vi "fp display engine.vi"(7 "channel data in":sgl[][][](array[numeric]), 10 "Image Refs In":T1[](array[typedef]), 11 "DisplayRefsIn(generic class)":refnum<vi>[](array[refnum])) -> ()   [LabVIEW 2012]
uses:
  <vilib>/vision/Image Controls.llb/IMAQ Image.ctl
  Custom Controls/MAIN Image panel tab Control type def.ctl
  Custom Controls/Ch selector.ctl
  GFG/GFGfpRefGet.vi
  GFG/GFGbooleanGet.vi
  <vilib>/vision/NI_Vision_Development_Module.lvlib
  GFG/GFG library.lvlib
panel:
  in  "ROI colors":u32[](array[colorbox])=[6618880, 16716362, 16860, 16776793, 16750848, 16448250, 16716530, 9567230, 16764108, 7340212, 32639, 0, 13816530, 8421376, 8421631, 7171459, 6618880, 16716362, 16860, 16776793, 16750848, 16448250, 16716530, 9567230, 16764108, 7340212, 32639, 0, 13816530, 8421376, 8421631, 7171459, 6618880, 16716362, 16860, 16776793, 16750848, 16448250, 16716530, 9567230, 16764108, 7340212, 32639, 0, 13816530, 8421376, 8421631, 7171459, 6618880, 16716362, 16860, 16776793, 16750848, 16448250, 16716530, 9567230, 16764108, 7340212, 32639, 0, 13816530, 8421376, 8421631, 7171459, 6618880, 16716362, 16860, 16776793, 16750848, 16448250, 16716530, 9567230, 16764108, 7340212, 32639, 0, 13816530, 8421376, 8421631, 7171459, 6618880, 16716362, 16860, 16776793, 16750848, 16448250, 16716530, 9567230, 16764108, 7340212, 32639, 0, 13816530, 8421376, 8421631, 7171459, 6618880, 16716362, 16860, 16776793, 16750848, 16448250, 16716530, 9567230, 16764108, 7340212, 32639, 0, 13816530, 8421376, 8421631, 7171459, 6618880, 16716362, 16860, 16776793, 16750848, 16448250, 16716530, 9567230, 16764108, 7340212, 32639, 0, 13816530, 8421376, 8421631, 7171459, 6618880, 16716362, 16860, 16776793, 16750848, 16448250, 16716530, 9567230, 16764108, 7340212, 32639, 0, 13816530, 8421376, 8421631, 7171459, 6618880, 16716362, 16860, 16776793, 16750848, 16448250, 16716530, 9567230, 16764108, 7340212, 32639, 0, 13816530, 8421376, 8421631, 7171459, 6618880, 16716362, 16860, 16776793, 16750848, 16448250, 16716530, 9567230, 16764108, 7340212, 32639, 0, 13816530, 8421376, 8421631, 7171459, 6618880, 16716362, 16860, 16776793, 16750848, 16448250, 16716530, 9567230, 16764108, 7340212, 32639, 0, 13816530, 8421376, 8421631, 7171459, 6618880, 16716362, 16860, 16776793, 16750848, 16448250, 16716530, 9567230, 16764108, 7340212, 32639, 0, 13816530, 8421376, 8421631, 7171459, 6618880, 16716362, 16860, 16776793, 16750848, 16448250, 16716530, 9567230, 16764108, 7340212, 32639, 0, 13816530, 8421376, 8421631, 7171459, 6618880, 16716362, 16860, 16776793, 16750848, 16448250, 16716530, 9567230, 16764108, 7340212, 32639, 0, 13816530, 8421376, 8421631, 7171459, 6618880, 16716362, 16860, 16776793, 16750848, 16448250, 16716530, 9567230, 16764108, 7340212, 32639, 0, 13816530, 8421376, 8421631, 7171459, 6618880, 16716362, 16860, 16776793, 16750848, 16448250, 16716530, 9567230, 16764108, 7340212, 32639, 0, 13816530, 8421376, 8421631, 7171459, 6618880, 16716362, 16860, 16776793, 16750848, 16448250, 16716530, 9567230, 16764108, 7340212, 32639, 0, 13816530, 8421376, 8421631, 7171459, 6618880, 16716362, 16860, 16776793, 16750848, 16448250, 16716530, 9567230, 16764108, 7340212, 32639, 0, 13816530, 8421376, 8421631, 7171459, 6618880, 16716362, 16860, 16776793, 16750848, 16448250, 16716530, 9567230, 16764108, 7340212, 32639, 0, 13816530, 8421376, 8421631, 7171459, 6618880, 16716362, 16860, 16776793, 16750848, 16448250, 16716530, 9567230, 16764108, 7340212, 32639, 0, 13816530, 8421376, 8421631, 7171459, 6618880, 16716362, 16860, 16776793, 16750848, 16448250, 16716530, 9567230, 16764108, 7340212, 32639, 0, 13816530, 8421376, 8421631, 7171459, 6618880, 16716362, 16860, 16776793, 16750848, 16448250, 16716530, 9567230, 16764108, 7340212, 32639, 0, 13816530, 8421376, 8421631, 7171459, 6618880, 16716362, 16860, 16776793, 16750848, 16448250, 16716530, 9567230, 16764108, 7340212, 32639, 0, 13816530, 8421376, 8421631, 7171459, 6618880, 16716362, 16860, 16776793, 16750848, 16448250, 16716530, 9567230, 16764108, 7340212, 32639, 0, 13816530, 8421376, 8421631, 7171459]
  out "error out":errorcluster
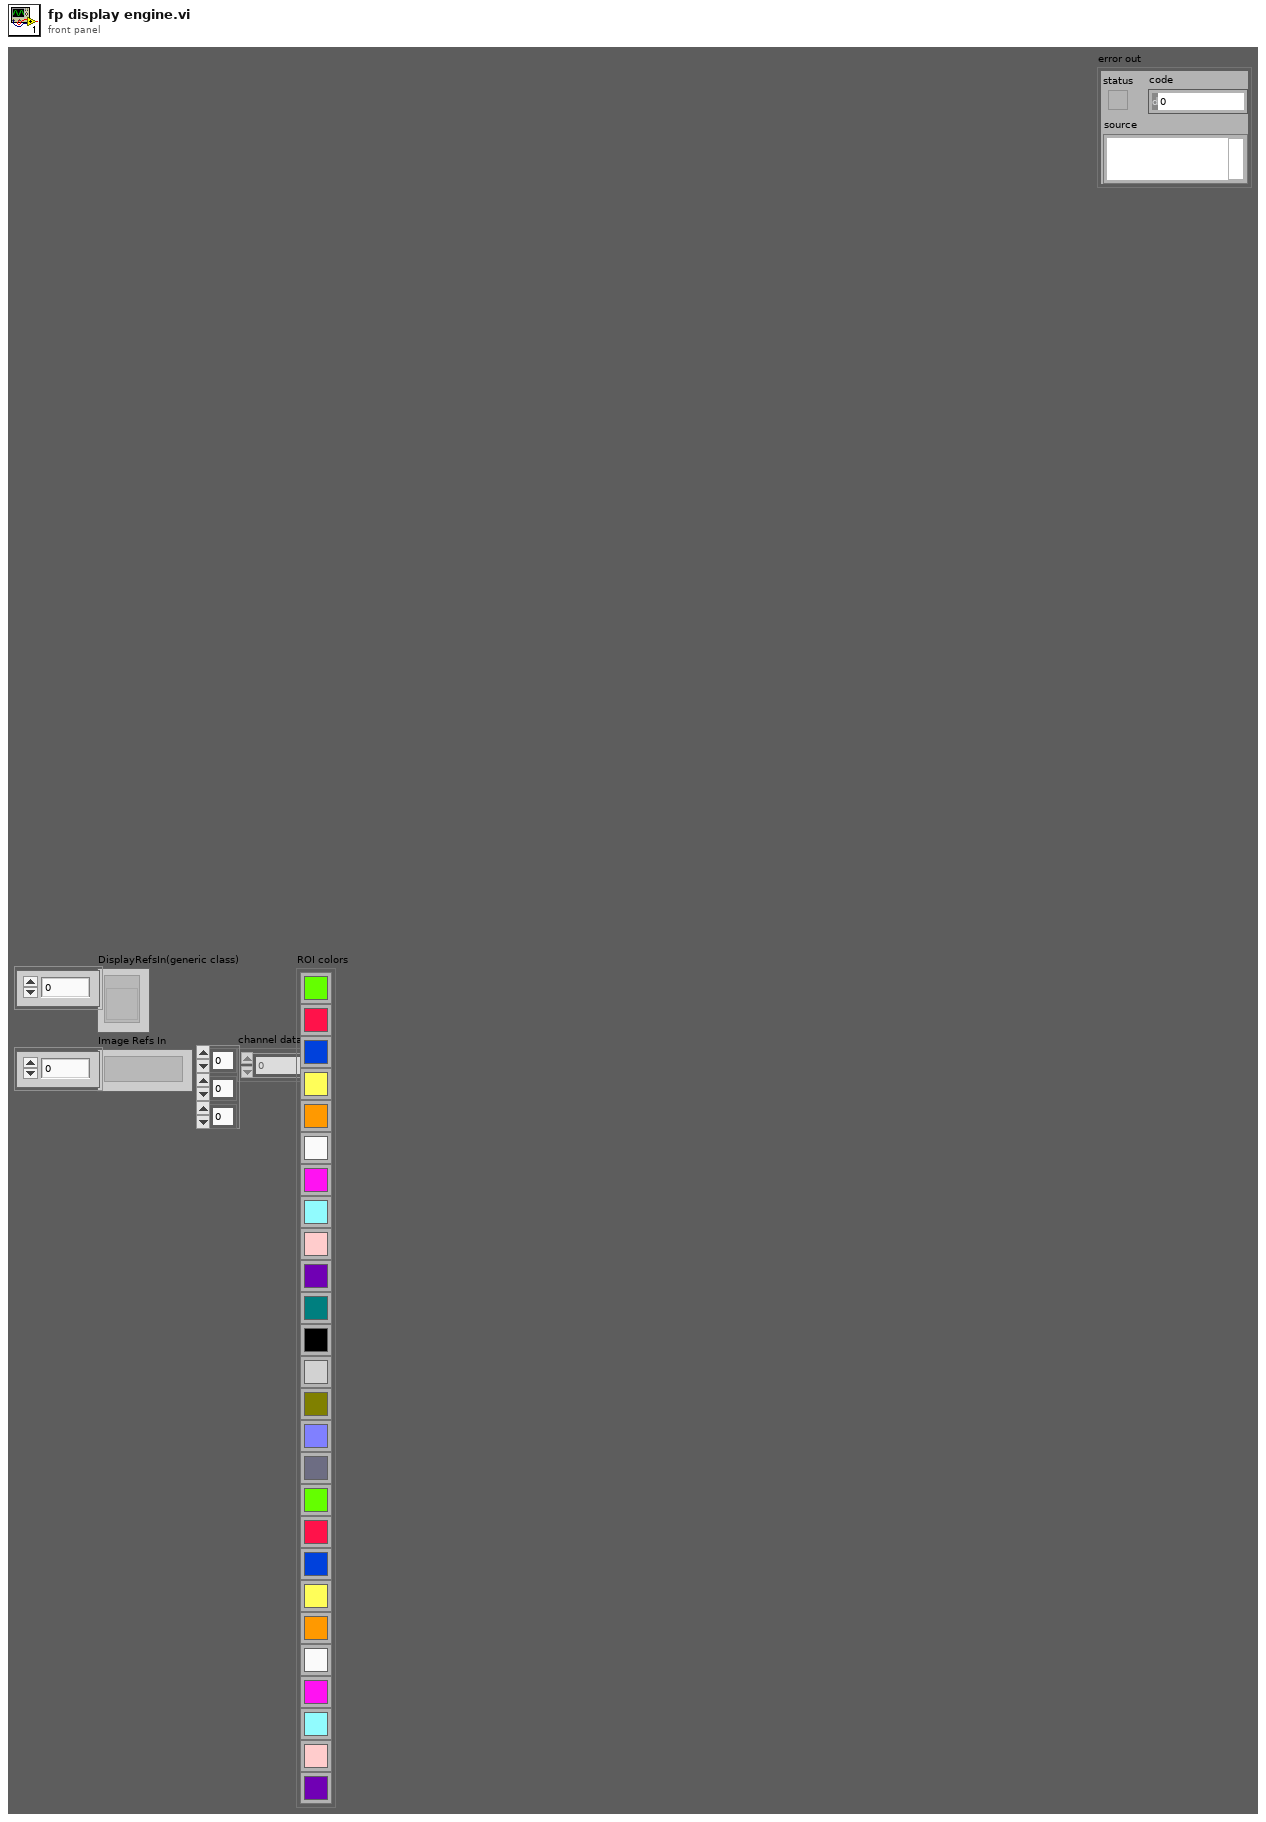
[diagram p1: front panel]
types:
  T1 = typedef "IMAQ Image.ctl" = refnum<image>
  T2 = typedef "MAIN Image panel tab Control type def.ctl" = enum32{"Channel 1", "Channel 2", "Channel 3", "Channel 4", "all channels", "RGB overlay", "ROI", "arbitrary line scan"}
  T3 = enum32{"Channel 1", "Channel 2", "Channel 3", "Channel 4", "Channel 5", "all channels", "RGB overlay", "ROI", "arbitrary line scan"}
  T4 = typedef "Ch selector.ctl" = enum16{"none", "Ch 1", "Ch 2", "Ch 3", "Ch 4", "Ch 5"}
  T5 = typedef "Image Type" = u32
  T6 = cluster{"Global Rectangle":i32[], "Contours":cluster{"Contour Type":u32, "ROI Type":u32, "Points":i32[]}[]}
  T7 = typedef "ROI Descriptor" = cluster{"Global Rectangle":i32[], "Contours":cluster{"ID":enum32{"External", "Internal"}, "Type":u32, "Coordinates":i32[]}[]}
  T8 = cluster{"WaveformChartRef":refnum<vi>, "DigitalRef":refnum<vi>, "ArrayRef":refnum<vi>, "TabControlRef":refnum<vi>, "EnumRef":refnum<vi>, "RingRef":refnum<vi>, "BooleanRef":refnum<vi>, "KnobRef":refnum<vi>, "SlideRef":refnum<vi>, "PathRef":refnum<vi>, "StringRef":refnum<vi>, "ComboBox":refnum<vi>, "WaveformGraphRef":refnum<vi>}
  T9 = cluster{"Mean Value":sgl, "Standard Variation":sgl, "Minimal Value":sgl, "Maximal Value":sgl, "Area (calibrated)":sgl, "Area (pixels)":i32, "%":sgl}[]
  T10 = cluster{"Mean Value":sgl, "Standard Variation":sgl, "Minimal Value":sgl, "Maximal Value":sgl, "Area (calibrated)":sgl, "Area (pixels)":i32, "%":sgl}
  T11 = cluster{"Contour Type":u32, "ROI Type":u32, "Points":i32[]}[]
  T12 = cluster{"Starting Value":sgl, "Incremental Value":sgl, "Histogram":u32[]}
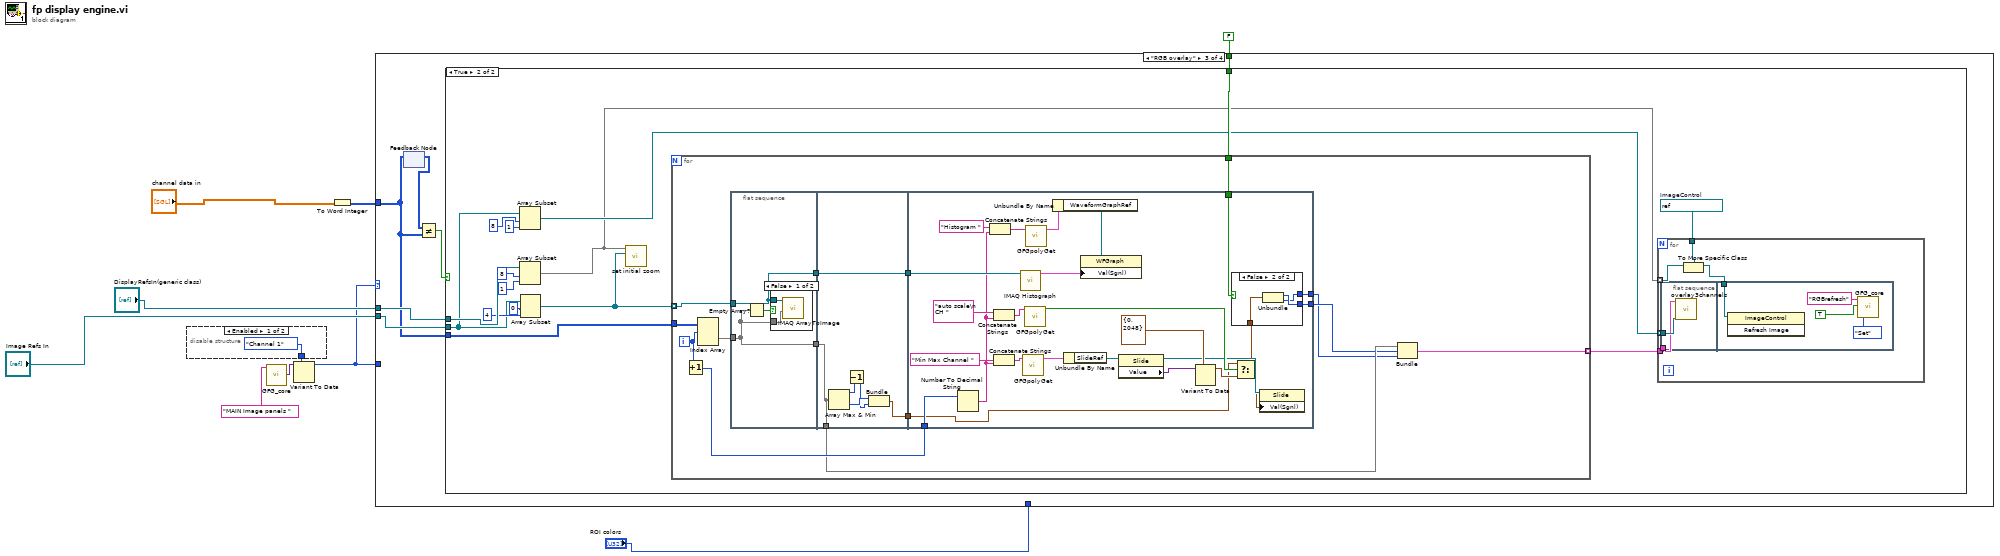
[diagram p0: block diagram]
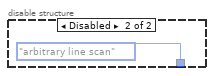
[diagram p2: hidden frame]
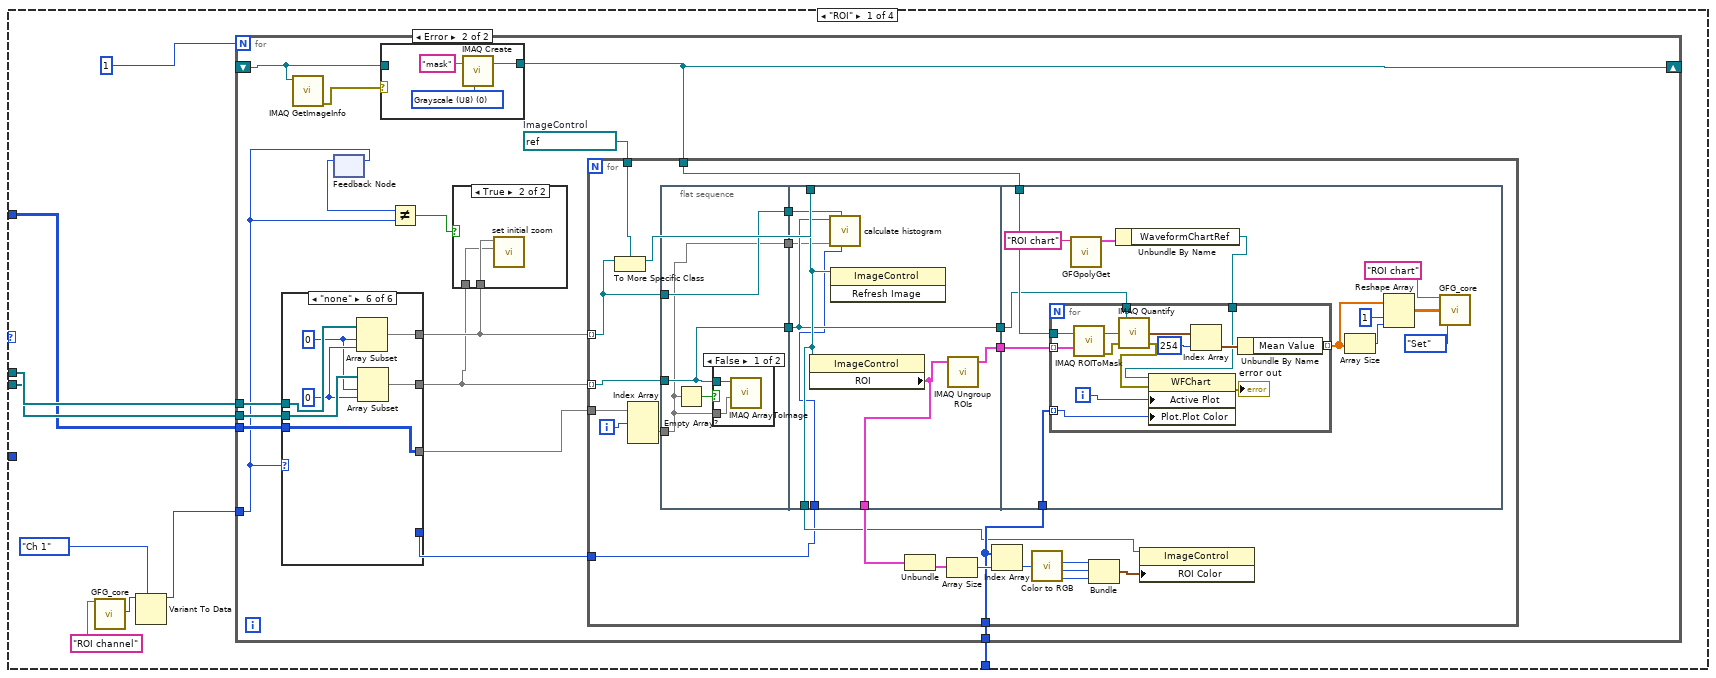
[diagram p3: hidden frame]
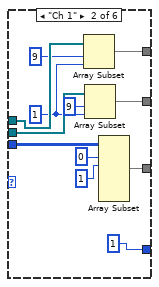
[diagram p7: hidden frame]
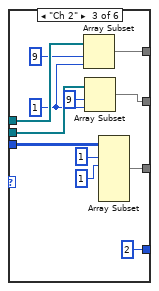
[diagram p8: hidden frame]
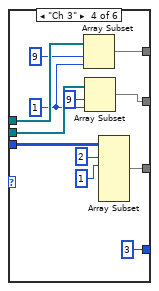
[diagram p9: hidden frame]
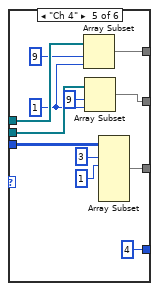
[diagram p10: hidden frame]
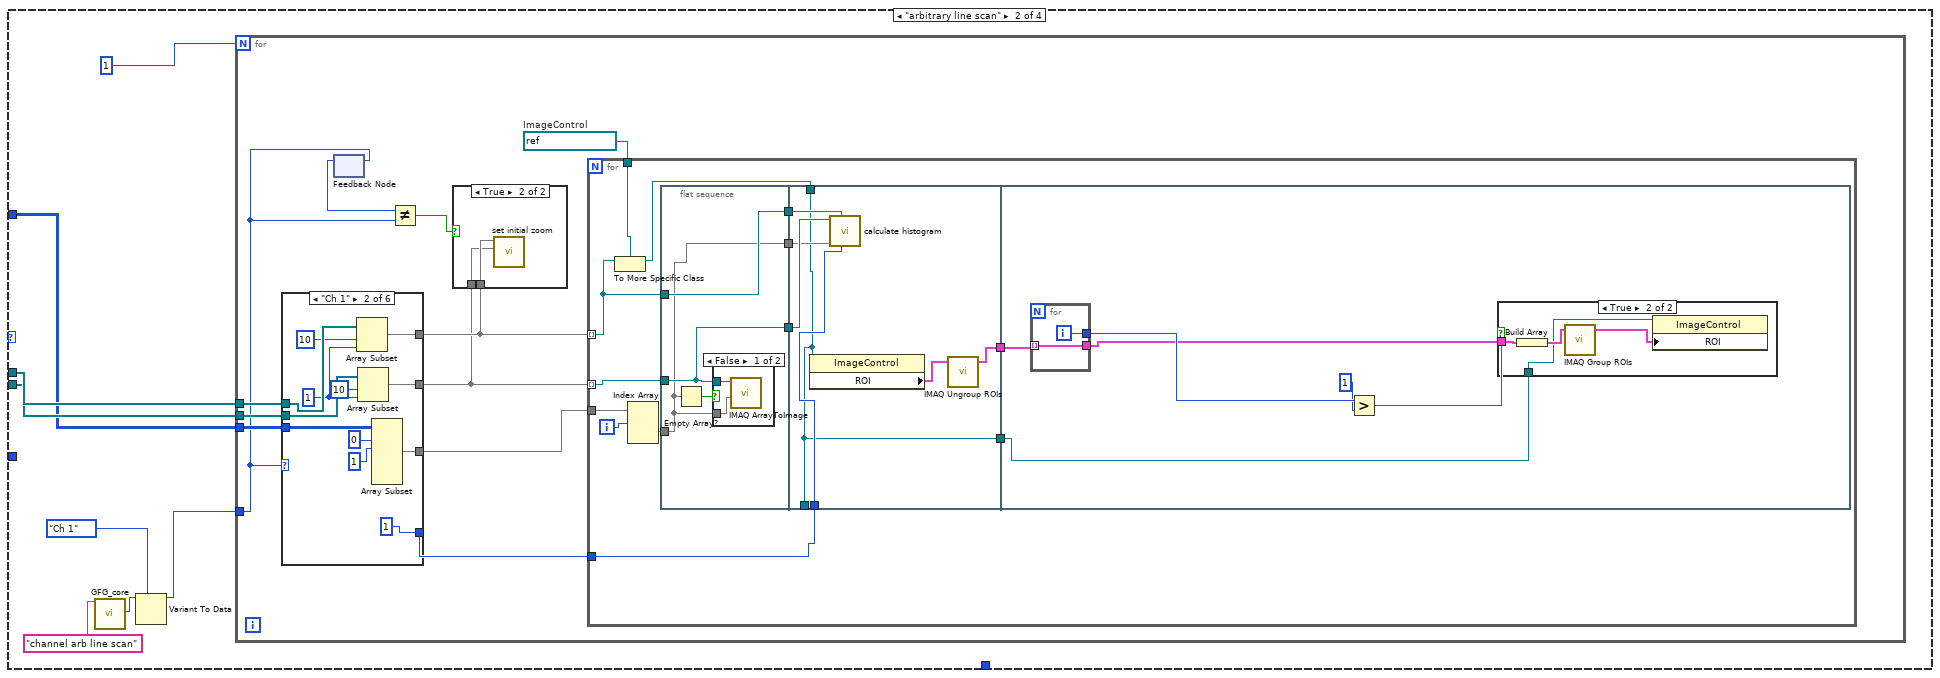
[diagram p12: hidden frame]
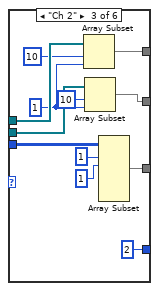
[diagram p15: hidden frame]
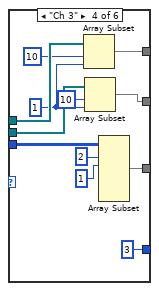
[diagram p16: hidden frame]
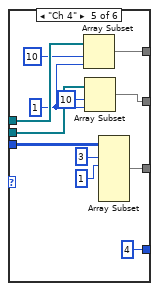
[diagram p17: hidden frame]
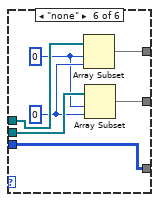
[diagram p18: hidden frame]
diagram:
  n1 = disable-structure shown="Enabled" {
    disable-tunnel: [MAIN_Image_panel_tab_Control_type_def."Channel 1" ("MAIN Image panels") T3."arbitrary line scan" ("MAIN Image panels")] -> w8
    frame Enabled {
    }
    frame Disabled {
    }
  }
  n2 = call "GFG_core.vi"("Variable Name in"="MAIN Image panels ") -> ("Variant Out"=w10:variant)  [unwired: 12 in, 6 out]
  n3 = Variant To Data(type=w8, Variant=w10) -> (data=w4:T2)  [unwired: 1 in, 1 out]
  n4 = To Word Integer(number="channel data in") -> (16bit integer=w3:i16[][][])
  n5 = case shown="\"RGB overlay\"" w4 {
    tunnel: w4 -> [_ _ _ w365]
    tunnel: "DisplayRefsIn(generic class)" -> [w20 w168 w281 w368]
    tunnel: "Image Refs In" -> [w19 w167 w279 w367]
    tunnel: w3 -> [w18 w166 w276 w366]
    tunnel: FALSE -> [_ _ w280 w363]
    tunnel: "ROI colors" -> [w14 _ _ _]
    frame "ROI" {
      n6 = call "GFG_core.vi"("Variable Name in"="ROI channel") -> ("Variant Out"=w16:variant)  [unwired: 12 in, 6 out]
      n7 = Variant To Data(type=Ch_selector."Ch 1" ("ROI channel"), Variant=w16) -> (data=w15:T4)  [unwired: 1 in, 1 out]
      n8 = for {
        N: 1 -> [_]
        tunnel: w20 -> [w35]
        tunnel: w19 -> [w34]
        tunnel: w18 -> [w33]
        tunnel: w15 -> [w30]
        shift-right: [w27] -> _
        shift-left: _ -> [w26]
        tunnel: w14 -> [w24]
        w32 = refnum<vi> refnum  # ImageControl
        n9 = case shown="\"none\"" w30 {
          tunnel: w35 -> [_ w53 w65 w77 w89 w96]
          tunnel: w34 -> [_ w54 w66 w78 w90 w97]
          tunnel: [_ w50 w62 w74 w86 w93] -> w22
          tunnel: [_ w49 w61 w73 w85 w92] -> w29
          tunnel: w33 -> [_ w48 w58 w70 w82 w91]
          tunnel: [_ w45 w57 w69 w81 w91] -> w36
          tunnel: [_ 1 ("length") 2 ("length") 3 ("length") 4 ("length") _] -> w23
          frame Default {
          }
          frame "Ch 1" {
            w52 = 1 ("length")
            n10 = Array Subset(array=w53, index=9, length=w52) -> (w49:refnum<vi>[])
            n11 = Array Subset(array=w54, index=9, length=w52) -> (w50:T1[])
            n12 = Array Subset(array=w48, index (dim 0)=0 ("index"), length (dim 0)=1 ("length")) -> (w45:i16[][][])  [unwired: 4 in]
          }
          frame "Ch 2" {
            w64 = 1 ("length")
            n13 = Array Subset(array=w65, index=9, length=w64) -> (w61:refnum<vi>[])
            n14 = Array Subset(array=w66, index=9, length=w64) -> (w62:T1[])
            n15 = Array Subset(array=w58, index (dim 0)=1 ("index"), length (dim 0)=1 ("length")) -> (w57:i16[][][])  [unwired: 4 in]
          }
          frame "Ch 3" {
            w75 = 1 ("index")
            n16 = Array Subset(array=w77, index=9, length=w75) -> (w73:refnum<vi>[])
            n17 = Array Subset(array=w78, index=9, length=w75) -> (w74:T1[])
            n18 = Array Subset(array=w70, index (dim 0)=2 ("index"), length (dim 0)=1 ("length")) -> (w69:i16[][][])  [unwired: 4 in]
          }
          frame "Ch 4" {
            w88 = 1 ("index")
            n19 = Array Subset(array=w89, index=9, length=w88) -> (w85:refnum<vi>[])
            n20 = Array Subset(array=w90, index=9, length=w88) -> (w86:T1[])
            n21 = Array Subset(array=w82, index (dim 0)=3 ("index"), length (dim 0)=1 ("length")) -> (w81:i16[][][])  [unwired: 4 in]
          }
          frame "none" {
            w94 = 0 ("index")
            w95 = 0 ("length")
            n22 = Array Subset(array=w96, index=w94, length=w95) -> (w92:refnum<vi>[])
            n23 = Array Subset(array=w97, index=w94, length=w95) -> (w93:T1[])
          }
        }
        n24 = call "IMAQ GetImageInfo"("Image"=w26) -> ("error out"=w25:errorcluster)  [unwired: 3 in, 7 out]
        n25 = feedback-in #1(w30) -> ()
        n26 = feedback #1() -> (w31:T4)  [unwired: 1 in]
        n27 = case shown="Error" w25 {
          tunnel: [w37 w38] -> w27
          tunnel: w26 -> [w37 _]
          frame No Error {
          }
          frame Error {
            w39 = T5 0 items=["Grayscale (U8)", "Grayscale (I16)", "Grayscale (SGL)", "Complex (CSG)", "RGB (U32)", "HSL (U32)", "RGB (U64)"] ("Image Type")
            n28 = call "IMAQ Create"("Image Name"="mask", "Image Type"=w39) -> ("New Image"=w38:T1)  [unwired: 3 in, 1 out]
          }
        }
        n29 = Not Equal?(x=w31, y=w30) -> (x != y?=w28:bool)
        n30 = case shown="True" w28 {
          tunnel: w29 -> [_ w42]
          tunnel: w22 -> [_ w41]
          frame False {
          }
          frame True {
            n31 = call "set initial zoom.vi"("Image Refs In"=w41, "DisplayRefsIn(generic class)"=w42) -> ()  [unwired: 10 in]
          }
        }
        n32 = for {
          tunnel: w29 -> [w100] mode=indexing
          tunnel: w22 -> [w119] mode=indexing
          tunnel: w36 -> [w121]
          tunnel: w32 -> [w118]
          tunnel: w27 -> [w103]
          tunnel: w24 -> [w106]
          tunnel: w23 -> [w98]
          i -> [w116]
          n33 = To More Specific Class(target class=w118, reference=w100) -> (specific class reference=w117:refnum<vi>)  [unwired: 1 in, 1 out]
          n34 = Index Array(array=w121, index (dim 0)=w116) -> (element=w120:i16[][])  [unwired: 2 in]
          n35 = flat-sequence {
            tunnel: w120 -> [w122]
            tunnel: w119 -> [w124]
            tunnel: [w124] -> w104
            tunnel: [w123] -> w101
            tunnel: w100 -> [w123]
            tunnel: [w122] -> w99
            tunnel: w117 -> [w132]
            tunnel: [w134] -> w109
            tunnel: [w133] -> w107
            tunnel: [w130] -> w105
            tunnel: w104 -> [w130]
            tunnel: [w132] -> w102
            tunnel: w101 -> [w131]
            tunnel: w99 -> [w129]
            tunnel: w98 -> [w128]
            tunnel: w107 -> [w144]
            tunnel: w106 -> [w143]
            tunnel: w105 -> [w135]
            tunnel: w103 -> [w136]
            frame #0 {
              n36 = Empty Array?(array=w122) -> (empty?=w125:bool)
              n37 = case shown="False" w125 {
                tunnel: w124 -> [w127 _]
                tunnel: w122 -> [w126 _]
                frame False {
                  n38 = call "IMAQ ArrayToImage"("Image Pixels (I16)"=w126, "Image"=w127) -> ()  [unwired: 8 in, 2 out]
                }
                frame True {
                }
              }
            }
            frame #1 {
              n39 = property class="ImageControl"(reference=w132) -> ("ROI"=w134:T6)  [unwired: 1 in, 2 out]
              n40 = call "calculate histogram.vi"("channel no."=w128, "Image Ctrl Ref (as generic class)"=w131, "Image Array"=w129, "Image"=w130) -> ()  [unwired: 8 in]
              n41 = invoke class="ImageControl" method="Refresh Image"(reference=w132) -> ()  [unwired: 2 in, 3 out]
              n42 = call "IMAQ Ungroup ROIs"("ROI Descriptor"=w134) -> ("ROI Descriptors out"=w133:T7[])  [unwired: 3 in, 1 out]
            }
            frame #2 {
              n43 = call-poly "GFGpolyGet.vi"("Variable Name in"="ROI chart") -> ("output cluster"=w138:T8)  [unwired: 9 in, 1 out]
              n44 = Unbundle By Name(w138) -> ("WaveformChartRef"=w137:refnum<vi>)
              n45 = for {
                tunnel: w135 -> [w161]
                tunnel: w144 -> [w155] mode=indexing
                tunnel: [w157] -> w147 mode=indexing
                tunnel: w136 -> [w154]
                tunnel: w143 -> [w151] mode=indexing
                tunnel: w137 -> [w150]
                i -> [w152]
                n46 = call "IMAQ ROIToMask"("ROI Descriptor"=w155, "Image"=w154) -> ("error out"=w149:errorcluster, "Image Out"=w156:T1)  [unwired: 4 in, 1 out]
                n47 = call "IMAQ Quantify"("error in (no error)"=w149, "Image Mask"=w156, "Image"=w161) -> ("error out"=w148:errorcluster, "Region Reports"=w160:T9)  [unwired: 1 out]
                n48 = property on="Property Node" class="WFChart"(reference=w150, error in=w148, "Active Plot"=w152, "Plot.Plot Color"=w151) -> (error out=→"error out":errorcluster)  [unwired: 1 out]
                n49 = Index Array(array=w160, index=254) -> (element=w158:T10)
                n50 = Unbundle By Name(w158) -> ("Mean Value"=w157:sgl)
              }
              n51 = Array Size(array=w147) -> (size(s)=w146:i32)
              n52 = Reshape Array(w147, 1 ("dimension size"), w146) -> (w141:sgl[][])
              n53 = call "GFG_core.vi"("Variable Name in"="ROI chart", "Variant in"=w141, "Action"=enum16{"Init", "Set", "Get"}."Set") -> ()  [unwired: 10 in, 7 out]
            }
          }
          n54 = Unbundle(w109) -> ("Contours"=w114:T11)  [unwired: 1 out]
          n55 = Array Size(array=w114) -> (size(s)=w115:i32)
          n56 = Index Array(array=w106, index=w115) -> (element=w110:u32)
          n57 = call <vilib>:"Color to RGB.vi"("Color"=w110) -> ("R"=w111:u8, "G"=w112:u8, "B"=w113:u8)  [unwired: 1 out]
          n58 = Bundle("R"=w111, "G"=w112, "B"=w113) -> (w108:cluster{"R":u8, "G":u8, "B":u8})  [unwired: 1 in]
          n59 = property class="ImageControl"(reference=w102, "ROI Color"=w108) -> ()  [unwired: 1 in, 2 out]
        }
      }
    }
    frame "arbitrary line scan" {
      n60 = call "GFG_core.vi"("Variable Name in"="channel arb line scan") -> ("Variant Out"=w164:variant)  [unwired: 12 in, 6 out]
      n61 = Variant To Data(type=Ch_selector."Ch 1" ("ROI channel"), Variant=w164) -> (data=w163:T4)  [unwired: 1 in, 1 out]
      n62 = for {
        N: 1 -> [_]
        tunnel: w168 -> [w179]
        tunnel: w167 -> [w178]
        tunnel: w166 -> [w177]
        tunnel: w163 -> [w174]
        w176 = refnum<vi> refnum  # ImageControl
        n63 = case shown="\"Ch 1\"" w174 {
          tunnel: w179 -> [_ w193 w205 w217 w229 w236]
          tunnel: w178 -> [_ w194 w206 w218 w230 w237]
          tunnel: [_ w190 w202 w214 w226 w233] -> w170
          tunnel: [_ w189 w201 w213 w225 w232] -> w173
          tunnel: w177 -> [_ w188 w198 w210 w222 w231]
          tunnel: [_ w185 w197 w209 w221 w231] -> w180
          tunnel: [_ 1 ("length") 2 ("length") 3 ("length") 4 ("length") _] -> w171
          frame Default {
          }
          frame "Ch 1" {
            w192 = 1 ("length")
            n64 = Array Subset(array=w193, index=10, length=w192) -> (w189:refnum<vi>[])
            n65 = Array Subset(array=w194, index=10, length=w192) -> (w190:T1[])
            n66 = Array Subset(array=w188, index (dim 0)=0 ("index"), length (dim 0)=1 ("length")) -> (w185:i16[][][])  [unwired: 4 in]
          }
          frame "Ch 2" {
            w204 = 1 ("length")
            n67 = Array Subset(array=w205, index=10, length=w204) -> (w201:refnum<vi>[])
            n68 = Array Subset(array=w206, index=10, length=w204) -> (w202:T1[])
            n69 = Array Subset(array=w198, index (dim 0)=1 ("index"), length (dim 0)=1 ("length")) -> (w197:i16[][][])  [unwired: 4 in]
          }
          frame "Ch 3" {
            w215 = 1 ("index")
            n70 = Array Subset(array=w217, index=10, length=w215) -> (w213:refnum<vi>[])
            n71 = Array Subset(array=w218, index=10, length=w215) -> (w214:T1[])
            n72 = Array Subset(array=w210, index (dim 0)=2 ("index"), length (dim 0)=1 ("length")) -> (w209:i16[][][])  [unwired: 4 in]
          }
          frame "Ch 4" {
            w228 = 1 ("index")
            n73 = Array Subset(array=w229, index=10, length=w228) -> (w225:refnum<vi>[])
            n74 = Array Subset(array=w230, index=10, length=w228) -> (w226:T1[])
            n75 = Array Subset(array=w222, index (dim 0)=3 ("index"), length (dim 0)=1 ("length")) -> (w221:i16[][][])  [unwired: 4 in]
          }
          frame "none" {
            w234 = 0 ("index")
            w235 = 0 ("length")
            n76 = Array Subset(array=w236, index=w234, length=w235) -> (w232:refnum<vi>[])
            n77 = Array Subset(array=w237, index=w234, length=w235) -> (w233:T1[])
          }
        }
        n78 = feedback-in #2(w174) -> ()
        n79 = feedback #2() -> (w175:T4)  [unwired: 1 in]
        n80 = Not Equal?(x=w175, y=w174) -> (x != y?=w172:bool)
        n81 = case shown="True" w172 {
          tunnel: w173 -> [_ w182]
          tunnel: w170 -> [_ w181]
          frame False {
          }
          frame True {
            n82 = call "set initial zoom.vi"("Image Refs In"=w181, "DisplayRefsIn(generic class)"=w182) -> ()  [unwired: 10 in]
          }
        }
        n83 = for {
          tunnel: w173 -> [w241] mode=indexing
          tunnel: w170 -> [w248] mode=indexing
          tunnel: w180 -> [w250]
          tunnel: w176 -> [w247]
          tunnel: w171 -> [w239]
          i -> [w245]
          n84 = To More Specific Class(target class=w247, reference=w241) -> (specific class reference=w246:refnum<vi>)  [unwired: 1 in, 1 out]
          n85 = Index Array(array=w250, index (dim 0)=w245) -> (element=w249:i16[][])  [unwired: 2 in]
          n86 = flat-sequence {
            tunnel: w249 -> [w251]
            tunnel: w248 -> [w253]
            tunnel: [w253] -> w243
            tunnel: [w252] -> w242
            tunnel: w241 -> [w252]
            tunnel: [w251] -> w240
            tunnel: w246 -> [w258]
            tunnel: [w263] -> w244
            tunnel: w243 -> [w261]
            tunnel: [w258] -> _
            tunnel: w242 -> [w262]
            tunnel: w240 -> [w260]
            tunnel: w239 -> [w259]
            tunnel: [w258] -> w238
            tunnel: w244 -> [w269]
            tunnel: w238 -> [w268]
            frame #0 {
              n87 = Empty Array?(array=w251) -> (empty?=w254:bool)
              n88 = case shown="False" w254 {
                tunnel: w253 -> [w256 _]
                tunnel: w251 -> [w255 _]
                frame False {
                  n89 = call "IMAQ ArrayToImage"("Image Pixels (I16)"=w255, "Image"=w256) -> ()  [unwired: 8 in, 2 out]
                }
                frame True {
                }
              }
            }
            frame #1 {
              n90 = property class="ImageControl"(reference=w258) -> ("ROI"=w257:T6)  [unwired: 1 in, 2 out]
              n91 = call "calculate histogram.vi"("channel no."=w259, "Image Ctrl Ref (as generic class)"=w262, "Image Array"=w260, "Image"=w261) -> ()  [unwired: 8 in]
              n92 = call "IMAQ Ungroup ROIs"("ROI Descriptor"=w257) -> ("ROI Descriptors out"=w263:T7[])  [unwired: 3 in, 1 out]
            }
            frame #2 {
              n93 = for {
                tunnel: w269 -> [w275] mode=indexing
                tunnel: [w275] -> w264
                tunnel: [w274] -> w267
                i -> [w274]
              }
              n94 = Greater?(x=w267, y=1) -> (0:w265:bool)
              n95 = case shown="True" w265 {
                tunnel: w264 -> [_ w273]
                tunnel: w268 -> [_ w270]
                frame False {
                }
                frame True {
                  n96 = Build Array(w273) -> (w272:T7[])
                  n97 = call "IMAQ Group ROIs"("ROI Descriptors"=w272) -> ("ROI Descriptor out"=w271:T7)  [unwired: 3 in, 1 out]
                  n98 = property class="ImageControl"(reference=w270, "ROI"=w271) -> ()  [unwired: 1 in, 2 out]
                }
              }
            }
          }
        }
      }
    }
    frame "RGB overlay" {
      n99 = feedback #3() -> (w278:i16[][][])  [unwired: 1 in]
      n100 = feedback-in #3(w276) -> ()
      n101 = Not Equal?(x=w278, y=w276) -> (x != y?=w277:bool)
      n102 = case shown="True" w277 {
        tunnel: w281 -> [_ w296]
        tunnel: w276 -> [_ w295]
        tunnel: w280 -> [_ w294]
        tunnel: w279 -> [_ w287]
        frame False {
        }
        frame True {
          w282 = refnum<vi> refnum  # ImageControl
          n103 = Array Subset(array=w287, index=8, length=1) -> (w286:T1[])
          n104 = Array Subset(array=w296, index=8, length=1) -> (w283:refnum<vi>[])
          n105 = Array Subset(array=w287, index=0, length=4) -> (w284:T1[])
          n106 = call "set initial zoom.vi"("Image Refs In"=w284, "DisplayRefsIn(generic class)"=w283) -> ()  [unwired: 10 in]
          n107 = for {
            tunnel: w284 -> [w319] mode=indexing
            tunnel: w295 -> [w321]
            tunnel: w294 -> [w312]
            tunnel: [w308] -> w285 mode=indexing
            i -> [w316]
            n108 = Increment(x=w316) -> (x+1=w314:i32)
            n109 = Index Array(array=w321, index (dim 0)=w316) -> (element=w320:i16[][])  [unwired: 2 in]
            n110 = flat-sequence {
              tunnel: w320 -> [w322]
              tunnel: w319 -> [w323]
              tunnel: [w323] -> w317
              tunnel: [w322] -> w315
              tunnel: [w332] -> w318
              tunnel: w317 -> [w332]
              tunnel: w315 -> [w327]
              tunnel: [w330] -> w313
              tunnel: [w327] -> w311
              tunnel: w318 -> [w351]
              tunnel: w314 -> [w350]
              tunnel: w313 -> [w338]
              tunnel: w312 -> [w333]
              tunnel: [w335] -> w309
              tunnel: [w334] -> w310
              frame #0 {
                n111 = Empty Array?(array=w322) -> (empty?=w324:bool)
                n112 = case shown="False" w324 {
                  tunnel: w323 -> [w326 _]
                  tunnel: w322 -> [w325 _]
                  frame False {
                    n113 = call "IMAQ ArrayToImage"("Image Pixels (I16)"=w325, "Image"=w326) -> ()  [unwired: 8 in, 2 out]
                  }
                  frame True {
                  }
                }
              }
              frame #1 {
                n114 = Array Max & Min(array=w327) -> (max value=w331:i16, min value=w329:i16)  [unwired: 2 out]
                n115 = Decrement(x=w331) -> (x-1=w328:i16)
                n116 = Bundle(w329, w328) -> (w330:cluster{i16, i16})  [unwired: 1 in]
              }
              frame #2 {
                n117 = Number To Decimal String(number=w350) -> (decimal integer string=w345:string)  [unwired: 1 in]
                n118 = Concatenate Strings("Histogram " ("string"), w345) -> (w353:string)
                n119 = Concatenate Strings("auto scale\n      CH " ("Variable Name in"), w345) -> (w348:string)
                n120 = Concatenate Strings("Min Max Channel " ("Variable Name in"), w345) -> (w336:string)
                n121 = call "IMAQ Histograph"("Image"=w351) -> ("Histogram Graph"=w356:T12)  [unwired: 7 in, 3 out]
                n122 = call-poly "GFGpolyGet.vi"("Variable Name in"=w336) -> ("output cluster"=w347:T8)  [unwired: 9 in, 1 out]
                n123 = call-poly "GFGpolyGet.vi"("Variable Name in"=w348) -> ("Boolean"=w341:bool)  [unwired: 10 in]
                n124 = call-poly "GFGpolyGet.vi"("Variable Name in"=w353) -> ("output cluster"=w354:T8)  [unwired: 9 in, 1 out]
                n125 = Unbundle By Name(w354) -> ("WaveformGraphRef"=w355:refnum<vi>)
                n126 = Unbundle By Name(w347) -> ("SlideRef"=w344:refnum<vi>)
                n127 = property class="WFGraph"(reference=w355, "Val(Sgnl)"=w356) -> ()  [unwired: 1 in, 2 out]
                n128 = property class="Slide"(reference=w344) -> (reference out=w339:refnum<vi>, "Value"=w343:variant)  [unwired: 1 in, 1 out]
                n129 = Variant To Data(type=cluster{i32, i32} {0, 2048} ("channel1"), Variant=w343) -> (data=w340:cluster{i32, i32})  [unwired: 1 in, 1 out]
                n130 = Select(t=w338, s=w341, f=w340) -> (s? t:f=w337:cluster{i32, i32})
                n131 = case shown="False" w333 {
                  tunnel: w337 -> [w359 w362]
                  tunnel: [w358 w360] -> w335
                  tunnel: [w357 w361] -> w334
                  frame True {
                    n132 = Unbundle(w359) -> (w358:i32, w357:i32)
                  }
                  frame False {
                    n133 = Unbundle(w362) -> (w361:i32, w360:i32)
                  }
                }
                n134 = property class="Slide"(reference=w339, "Val(Sgnl)"=w337) -> ()  [unwired: 1 in, 2 out]
              }
            }
            n135 = Bundle(w311, w310, w309) -> (w308:cluster{i16[][], i32, i32})  [unwired: 1 in]
          }
          n136 = for {
            tunnel: w286 -> [w301] mode=indexing
            tunnel: w285 -> [w300]
            tunnel: w283 -> [w299] mode=indexing
            tunnel: w282 -> [w298]
            n137 = flat-sequence {
              tunnel: w301 -> [w303]
              tunnel: w300 -> [w302]
              tunnel: w297 -> [w307]
              frame #0 {
                n138 = call "overlay3channels.vi"("RGB Overlay"=w303, "Array"=w302) -> ()  [unwired: 10 in]
              }
              frame #1 {
                n139 = invoke class="ImageControl" method="Refresh Image"(reference=w307) -> ()  [unwired: 2 in, 3 out]
                n140 = call "GFG_core.vi"("Variable Name in"="RGBrefresh", "Variant in"=TRUE, "Action"=enum16{"Init", "Set", "Get"}."Set") -> ()  [unwired: 10 in, 7 out]
              }
            }
            n141 = To More Specific Class(target class=w298, reference=w299) -> (specific class reference=w297:refnum<vi>)  [unwired: 1 in, 1 out]
          }
        }
      }
    }
    frame Default {
      n142 = for {
        N: 1 -> [_]
        tunnel: w368 -> [w378]
        tunnel: w367 -> [w377]
        tunnel: w366 -> [w376]
        tunnel: w365 -> [w371]
        tunnel: w363 -> [w373]
        shift-right: [w371] -> _
        shift-left: _ -> [w370]
        n143 = case shown="\"Channel 1\"" w371 {
          tunnel: w378 -> [_ w390 w400 w410 w420 w427]
          tunnel: w377 -> [_ w391 w401 w411 w421 w428]
          tunnel: [_ w387 w397 w407 w417 w424] -> w372
          tunnel: [_ w386 w396 w406 w416 w423] -> w375
          tunnel: w376 -> [_ w385 w393 w403 w413 w422]
          tunnel: [_ w382 w392 w402 w412 w422] -> w379
          frame Default {
          }
          frame "Channel 1" {
            w388 = 4 ("index")
            w389 = 1 ("length")
            n144 = Array Subset(array=w390, index=w388, length=w389) -> (w386:refnum<vi>[])
            n145 = Array Subset(array=w391, index=w388, length=w389) -> (w387:T1[])
            n146 = Array Subset(array=w385, index (dim 0)=0 ("index"), length (dim 0)=1 ("length")) -> (w382:i16[][][])  [unwired: 4 in]
          }
          frame "Channel 2" {
            w398 = 5 ("index")
            w399 = 1 ("length")
            n147 = Array Subset(array=w400, index=w398, length=w399) -> (w396:refnum<vi>[])
            n148 = Array Subset(array=w401, index=w398, length=w399) -> (w397:T1[])
            n149 = Array Subset(array=w393, index (dim 0)=1 ("index"), length (dim 0)=1 ("length")) -> (w392:i16[][][])  [unwired: 4 in]
          }
          frame "Channel 3" {
            w408 = 1 ("index")
            w409 = 6 ("index")
            n150 = Array Subset(array=w410, index=w409, length=w408) -> (w406:refnum<vi>[])
            n151 = Array Subset(array=w411, index=w409, length=w408) -> (w407:T1[])
            n152 = Array Subset(array=w403, index (dim 0)=2 ("index"), length (dim 0)=1 ("length")) -> (w402:i16[][][])  [unwired: 4 in]
          }
          frame "Channel 4" {
            w418 = 7 ("index")
            w419 = 1 ("index")
            n153 = Array Subset(array=w420, index=w418, length=w419) -> (w416:refnum<vi>[])
            n154 = Array Subset(array=w421, index=w418, length=w419) -> (w417:T1[])
            n155 = Array Subset(array=w413, index (dim 0)=3 ("index"), length (dim 0)=1 ("length")) -> (w412:i16[][][])  [unwired: 4 in]
          }
          frame "all channels" {
            w425 = 0 ("index")
            w426 = 4 ("length")
            n156 = Array Subset(array=w427, index=w425, length=w426) -> (w423:refnum<vi>[])
            n157 = Array Subset(array=w428, index=w425, length=w426) -> (w424:T1[])
          }
        }
        n158 = Not Equal?(x=w370, y=w371) -> (x != y?=w374:bool)
        n159 = for {
          tunnel: w375 -> [w431] mode=indexing
          tunnel: w372 -> [w433] mode=indexing
          tunnel: w379 -> [w438]
          tunnel: w371 -> [w437]
          tunnel: w373 -> [_]
          tunnel: [w430] -> w369
          i -> [w430]
          n160 = Increment(x=w430) -> (x+1=w436:i32)
          n161 = Index Array(array=w438, index (dim 0)=w430) -> (element=w432:i16[][])  [unwired: 2 in]
          n162 = flat-sequence {
            tunnel: w432 -> [w439]
            tunnel: w433 -> [w440]
            tunnel: [w440] -> w435
            tunnel: [w439] -> w434
            tunnel: w435 -> [w445]
            tunnel: w434 -> [w447]
            tunnel: w429 -> [w446]
            tunnel: w431 -> [w444]
            frame #0 {
              n163 = Empty Array?(array=w439) -> (empty?=w441:bool)
              n164 = case shown="False" w441 {
                tunnel: w440 -> [w443 _]
                tunnel: w439 -> [w442 _]
                frame False {
                  n165 = call "IMAQ ArrayToImage"("Image Pixels (I16)"=w442, "Image"=w443) -> ()  [unwired: 8 in, 2 out]
                }
                frame True {
                }
              }
            }
            frame #1 {
              n166 = call "calculate histogram.vi"("channel no."=w446, "Image Ctrl Ref (as generic class)"=w444, "Image Array"=w447, "Image"=w445) -> ()  [unwired: 8 in]
            }
          }
          n167 = case shown="\"all channels\"" w437 {
            tunnel: [1 2 3 4 w452] -> w429
            tunnel: w436 -> [_ _ _ _ w452]
            frame "Channel 1", Default {
            }
            frame "Channel 2" {
            }
            frame "Channel 3" {
            }
            frame "Channel 4" {
            }
            frame "all channels" {
            }
          }
        }
        n168 = case shown="True" w374 {
          tunnel: w375 -> [_ w381]
          tunnel: w372 -> [_ w380]
          tunnel: w369 -> [_ _]
          frame False {
          }
          frame True {
            n169 = call "set initial zoom.vi"("Image Refs In"=w380, "DisplayRefsIn(generic class)"=w381) -> ()  [unwired: 10 in]
          }
        }
      }
    }
  }
